vi "LVFunction_Imop_GetSDKConfig.vi"(0 "Configuration file path":path, 11 "error in":errorcluster) -> (4 "has_haso_sdk":bool, 6 "has_casao_sdk":bool, 8 "has_options_sdk":bool, 10 "has_x64_traitepente":bool, 15 "error out":errorcluster)   [LabVIEW 2018]
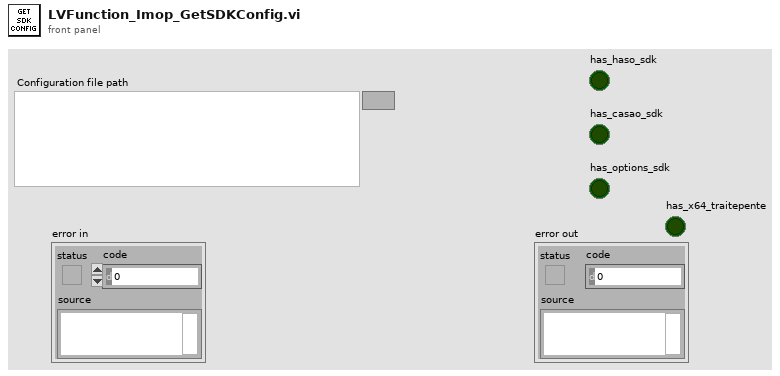
[diagram p1: front panel]
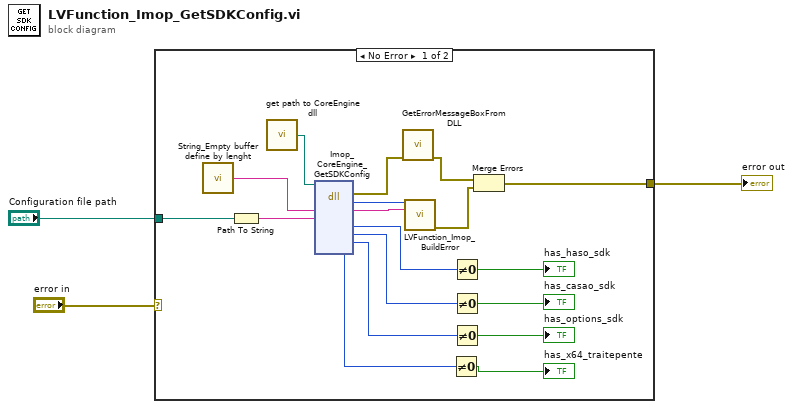
[diagram p0: block diagram]
diagram:
  n1 = case shown="No Error" "error in" {
    selector: "error in" -> [_ w22]
    tunnel: [w14 w22] -> w2
    tunnel: "Configuration file path" -> [w13 _]
    frame No Error {
      n2 = call "String_Empty buffer define by lenght.vi"() -> ("Empty buffer"=w15:string)  [unwired: 1 in]
      n3 = Path To String(path=w13) -> (string=w12:string)
      n4 = call "get path to CoreEngine dll.vi"() -> ("path to wavekit library"=w18:path)  [unwired: 14 in, 1 out]
      n5 = dll-call lib="D:/soft/HASO_v3/SVN_trunk/ImOpCoreEngine4_LV2011/DLLs/c_interface_vc100.dll" fn="Imop_CoreEngine_GetSDKConfig"(path in=w18, "message"=w15, "config_file_path"=w12) -> (error out=w19:errorcluster, "return type"=w17:i32, "message"=w16:string, "has_haso_sdk"=w11:u8, "has_casao_sdk"=w10:u8, "has_options_sdk"=w5:u8, "has_x64_traitepente"=w6:u8)  [unwired: 7 in, 1 out]
      n6 = call "GetErrorMessageBoxFromDLL.vi"("error IN"=w19) -> ("error OUT"=w20:errorcluster)  [unwired: 10 in]
      n7 = call "LVFunction_Imop_BuildError.vi"("code"=w17, "String to Prepend to source (\"\")"=w16) -> ("error out"=w21:errorcluster)  [unwired: 13 in]
      n8 = Not Equal To 0?(x=w6) -> (x != 0?=→"has_x64_traitepente":bool)
      n9 = Not Equal To 0?(x=w11) -> (x != 0?=→"has_haso_sdk":bool)
      n10 = Not Equal To 0?(x=w10) -> (x != 0?=→"has_casao_sdk":bool)
      n11 = Not Equal To 0?(x=w5) -> (x != 0?=→"has_options_sdk":bool)
      n12 = Merge Errors(w20, w21) -> (w14:errorcluster)
    }
    frame Error {
    }
  }
  "error out" <- w2
